vi "Imaging Data Address Control.vi"(11 "Imaging data displayed":u32) -> (3 "Clean":bool)   [LabVIEW 2015]
uses:
  OpenScan Labview code_20170126/Global_Sample per Frame.vi
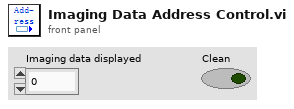
[diagram p1: front panel]
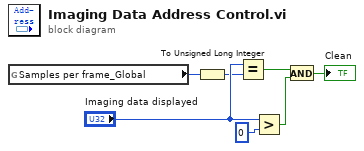
[diagram p0: block diagram]
diagram:
  n1 = global read "Global_Sample per Frame.vi" "Samples per frame_Global"() -> (w5:u32)
  n2 = To Unsigned Long Integer(number=w5) -> (unsigned 32bit integer=w1:u32)
  n3 = Equal?(x="Imaging data displayed", y=w1) -> (x = y?=w4:bool)
  n4 = Greater?(x="Imaging data displayed", y=u32 0) -> (0:w3:bool)
  n5 = And(x=w4, y=w3) -> (x .and. y?=→"Clean":bool)
